vi "Read_Single_chirp_Waveform.vi"(8 "error in (no error)":errorcluster, 9 "Maximum Time (10000 ms)":u32=10000, 11 "VISA resource name":refnum<visa-resource-name>) -> (0 "error out":errorcluster, 2 "Waveform Data":waveform(dbl)(graph), 3 "VISA resource name out":refnum<visa-resource-name>, 4 "curve & length command":u32, 5 "low level meas time":u32, 6 "fetch waveform timing":u32)   [LabVIEW 2011]
doc: "Initiates an acquisition on all channels that you enabled with the Configure Channel VI. This VI waits for the acquisition to complete and returns the waveform for the <B>Channel</B> you specify. If the oscilloscope does not complete the acquisition within the <B>Maximum Time</B> period, this VI returns a timeout error. A timeout error often occurs because the acquisition is not triggered. For example, if the trigger level is out of range of the waveform, the acquisition is not triggered.\n\nRun the Fetch Waveform VI to obtain the waveforms for each of the remaining enabled <B>Channels</B> without initiating another acquisition.\n\n<B>Note:</B> If the instrument does not support autocompensation for probe attenuation, you might need to adjust the scaling of the <B>Waveform Data</B> accordingly. You can adjust the scaling using the Configure Channel VI or manually multiplying the <B>Waveform Data</B> by the probe attenuation."
uses:
  <instrlib>/Tektronix 7000 Series/Tektronix 7000 Series.lvlib
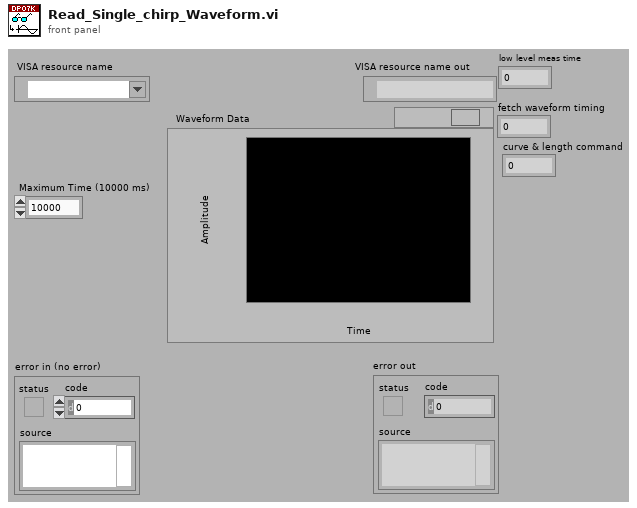
[diagram p1: front panel]
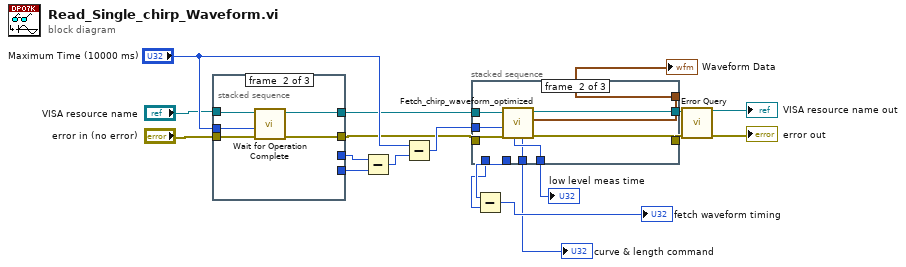
[diagram p0: block diagram]
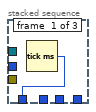
[diagram p2: hidden frame]
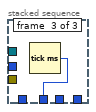
[diagram p3: hidden frame]
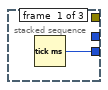
[diagram p4: hidden frame]
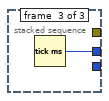
[diagram p5: hidden frame]
diagram:
  n1 = stacked-sequence {
    tunnel: "VISA resource name" -> [_ w25 _]
    tunnel: "error in (no error)" -> [_ w24 _]
    tunnel: [_ _ w26] -> w14
    tunnel: [w20 _ _] -> w13
    tunnel: "Maximum Time (10000 ms)" -> [_ w23 _]
    tunnel: [_ w22 _] -> w9
    tunnel: [_ w21 _] -> w8
    frame #0 {
      n2 = Tick Count (ms)() -> (millisecond timer value=w20:u32)
    }
    frame #1 {
      n3 = call <instrlib>:"Wait for Operation Complete.vi"("error in (no error)"=w24, "Maximum Time (2000ms)"=w23, "VISA resource name"=w25) -> ("error out"=w21:errorcluster, "VISA resource name out"=w22:refnum<visa-resource-name>)  [unwired: 7 in]
    }
    frame #2 {
      n4 = Tick Count (ms)() -> (millisecond timer value=w26:u32)
    }
  }
  n5 = Subtract(x=w14, y=w13) -> (x-y=w12:u32)
  n6 = Subtract(x="Maximum Time (10000 ms)", y=w12) -> (x-y=w10:u32)
  n7 = stacked-sequence {
    tunnel: [_ w35 _] -> w17
    tunnel: [_ w34 _] -> w16
    tunnel: [_ w33 _] -> w15
    tunnel: w10 -> [_ w32 _]
    tunnel: w9 -> [_ w31 _]
    tunnel: w8 -> [_ w30 _]
    tunnel: [w27 _ _] -> w4
    tunnel: [_ _ w36] -> w5
    tunnel: [_ w29 _] -> w2
    tunnel: [_ w28 _] -> w1
    frame #0 {
      n8 = Tick Count (ms)() -> (millisecond timer value=w27:u32)
    }
    frame #1 {
      n9 = call "Fetch_chirp_waveform_optimized.vi"("error in (no error)"=w30, "Maximum Time (10000ms)"=w32, "VISA resource name"=w31) -> ("error out"=w34:errorcluster, "Waveform Data"=w33:waveform(dbl), "VISA resource name out"=w35:refnum<visa-resource-name>, "curvea and length command"=w28:u32, "meas time"=w29:u32)  [unwired: 4 in]
    }
    frame #2 {
      n10 = Tick Count (ms)() -> (millisecond timer value=w36:u32)
    }
  }
  "Waveform Data" <- w15
  "low level meas time" <- w2
  "curve & length command" <- w1
  n11 = Subtract(x=w5, y=w4) -> (x-y=→"fetch waveform timing":u32)
  n12 = call <instrlib>:"Error Query.vi"("error in (no error)"=w16, "VISA resource name"=w17) -> ("error out"=→"error out":errorcluster, "VISA resource name out"=→"VISA resource name out":refnum<visa-resource-name>)  [unwired: 6 in, 2 out]
